vi "Configure Add Panel Control_Msg.vi"(8 "error in (no error)":errorcluster, 11 "Add Panel Control_Msg":refnum<class "Add Control_Behavior.lvclass">) -> (0 "error out":errorcluster, 3 "Add Panel Control_Msg Out":refnum<class "Add Control_Behavior.lvclass">)   [LabVIEW 2015, in "Add Control_Behavior.lvclass"]
doc: "This VI sends the message to an actor."
uses:
  Add Control_Behavior.lvclass
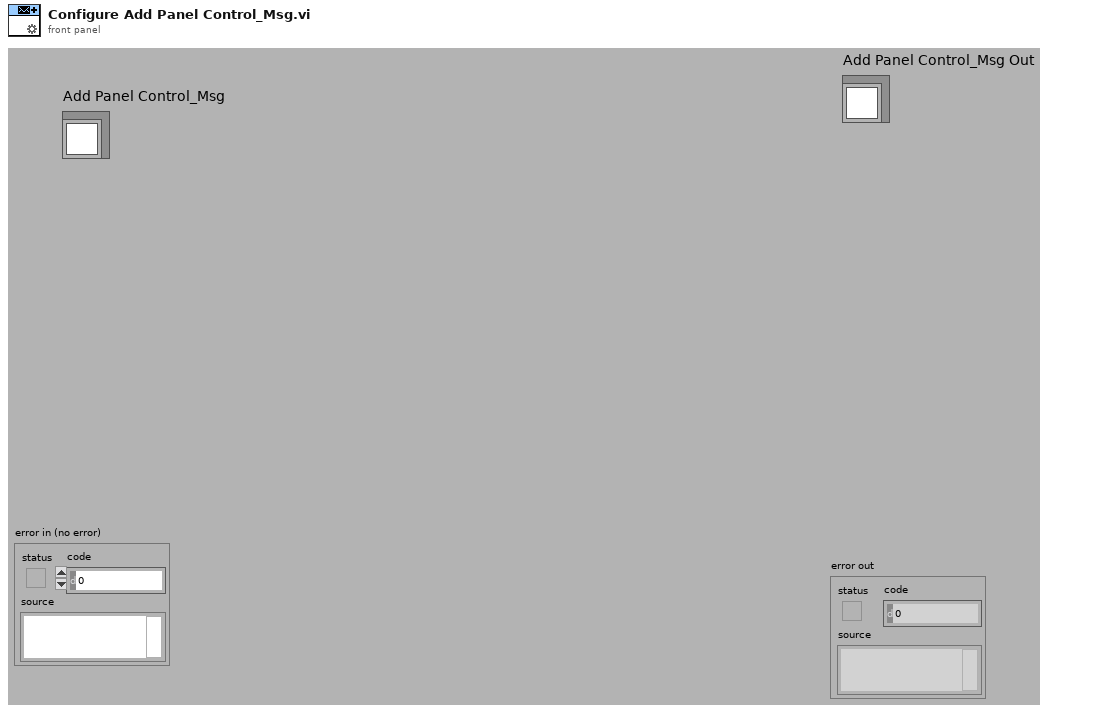
[diagram p1: front panel]
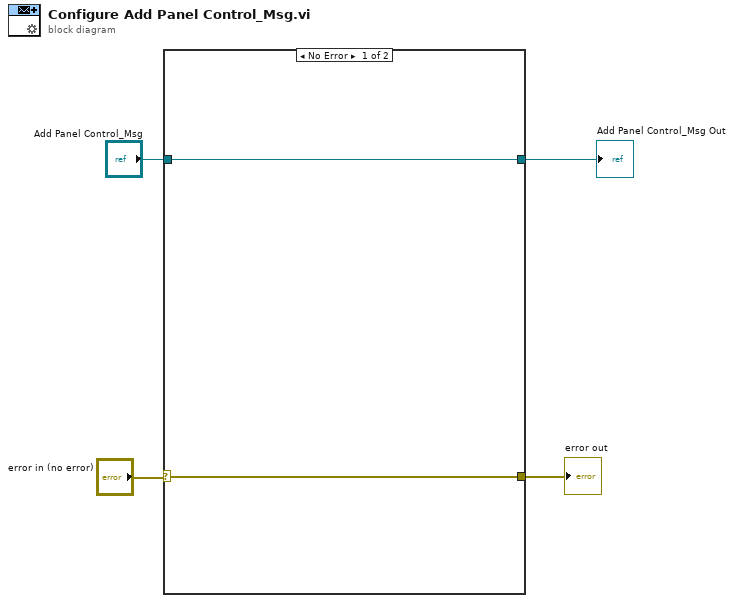
[diagram p0: block diagram]
diagram:
  n1 = case shown="No Error" "error in (no error)" {
    selector: "error in (no error)" -> [w6 w8]
    tunnel: "Add Panel Control_Msg" -> [w5 w7]
    tunnel: [w5 w7] -> w3
    tunnel: [w6 w8] -> w1
    frame No Error {
    }
    frame Error {
    }
  }
  "error out" <- w1
  "Add Panel Control_Msg Out" <- w3
